vi "FPGA Target AIO Example.vi"() -> ()   [LabVIEW 2021]
doc: "This example reads an AI port and writes to an AO port"
uses:
  <vilib>/rvi/Emulation/niFpgaGetClockAttributes.vi
  <vilib>/rvi/Emulation/niFpgaSctlEmulationGetInTimedLoop.vi
  <vilib>/rvi/Emulation/niFpgaEmulationReportErrorSimple.vi
  <vilib>/rvi/eio/common/nirviEmuTemplateMethod_errors.vi
  <vilib>/rvi/Emulation/niFpgaCriticalErrorInLSC.vi
  <vilib>/eio/EIONode/EIONode.xnode
panel:
  out "Connector0/AI0":i16
  in  "Connector0/AO0":i16
  # "*Connect AO0 to AI0 using the SCB-68 board (check pinout of the FPGA card because it is different from the E series devices.\nNote that every time you modify this VI, it will need to be recompiled."
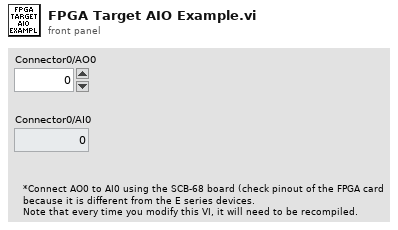
[diagram p1: front panel]
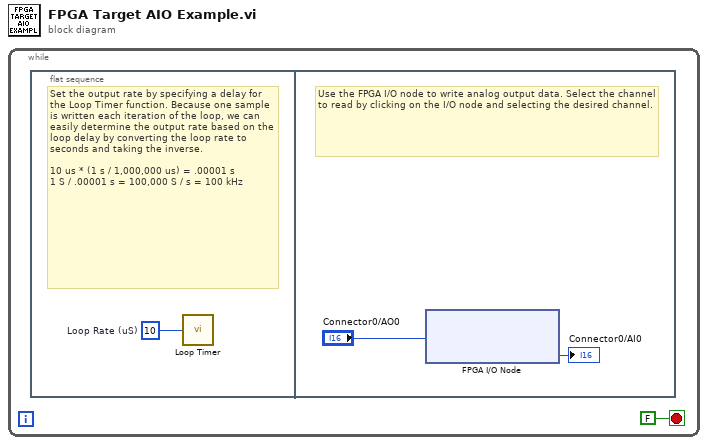
[diagram p0: block diagram]
diagram:
  n1 = while {
    stop <- FALSE ("Stop") stop-if-true
    # "Main Processing Loop"
    n2 = flat-sequence {
      frame #0 {
        w2 = u32 10  # Loop Rate (uS)
        # "Set the output rate by specifying a delay for the Loop Timer function. Because one sample is written each iteration of the loop, we can easily determine the output rate based on the loop delay by converting the loop rate to seconds and taking the inverse. \n\n10 us * (1 s / 1,000,000 us) = .00001 s\n1 S / .00001 s = 100,000 S / s = 100 kHz"
        n3 = call "Loop Timer"("Count(uSec)"=w2) -> ()  [unwired: 1 out]
      }
      frame #1 {
        # "Use the FPGA I/O node to write analog output data. Select the channel to read by clicking on the I/O node and selecting the desired channel."
        n4 = xnode "FPGA I/O Node"("Connector0/AO0"="Connector0/AO0") -> ("Connector0/AI0"=→"Connector0/AI0":i16)  [unwired: 2 in, 2 out]
      }
    }
  }
